vi "SW Interface - SET - Triggered Event.vi"(8 "error in (no error)":errorcluster, 10 "Events":T1, 11 "Child_2_Class in":refnum<class "SW_Interface_Class.lvclass">) -> (0 "error out":errorcluster, 3 "Child_2_Class out":refnum<class "SW_Interface_Class.lvclass">)   [LabVIEW 2023, in "SW_Interface_Actor.lvlib" / "SW_Interface_Class.lvclass"]
uses:
  SW_Interface_Class.lvclass
  Usr Ev/SW Interface - Ctrl - Enum - Events (Temp).ctl
  SW_Interface_Class.lvclass/SW_Interface_Class.ctl
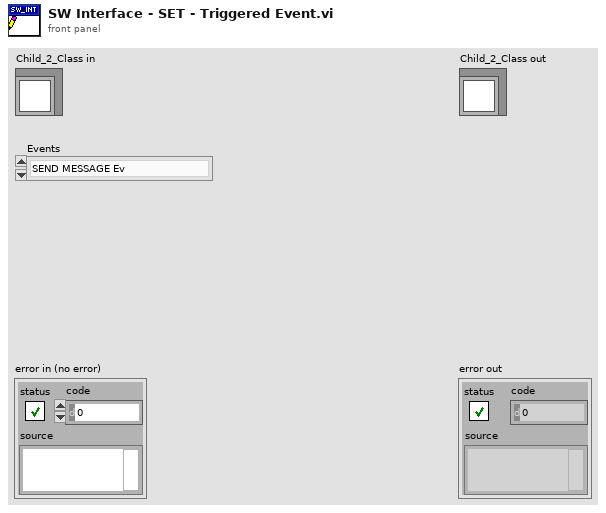
[diagram p1: front panel]
types:
  T1 = typedef "SW_Interface_Actor.lvlib/SW_Interface_Class.lvclass/SW Interface - Ctrl - Enum - Events (Temp).ctl" = enum16{"SEND MESSAGE Ev", "STOP_ACTOR Ev", "INIT_ACTOR Ev", "START Ev", "STOP Ev", "GET Ev", "SET Ev", "ERROR_HANDLER Ev", "RESET Ev", "T2 Ev", "T3 Ev", "T4 Ev"}
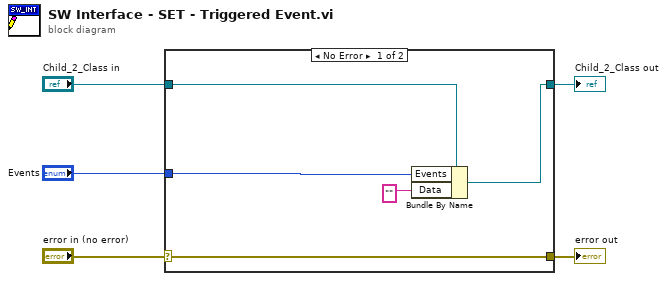
[diagram p0: block diagram]
diagram:
  n1 = case shown="No Error" "error in (no error)" {
    selector: "error in (no error)" -> [w10 w11]
    tunnel: [w10 w11] -> w4
    tunnel: [w8 w12] -> w2
    tunnel: "Child_2_Class in" -> [w9 w12]
    tunnel: "Events" -> [w7 _]
    frame No Error {
      n2 = Bundle By Name(cluster=w9, "Events"=w7, "Data"="") -> (w8:refnum<class "SW_Interface_Class.lvclass">)
    }
    frame Error {
    }
  }
  "error out" <- w4
  "Child_2_Class out" <- w2
